vi "Servos Module Testing.vi"(0 "Stop Button":bool) -> ()   [LabVIEW 2015]
uses:
  <vilib>/FPGAPlugInAG/myRIO-1900/niLvFpga_Open_myRIO-1900.vi
  <vilib>/rvi/interface/common/dynamic/niFpgaDynamicAddResources.vi
  <vilib>/FPGAPlugInAG/Dynamic/niLvFpga_Run_Dynamic.vi
  <vilib>/FPGAPlugInAG/Dynamic/niLvFpga_Close_Dynamic.vi
  <vilib>/rvi/interface/nirviOpenFPGA/nirviOpenFPGA.xnode
  FPGA Bitfiles/PDMSMain_FPGATarget-Wi-Fi_Express2_Jo8xc+hAvHc.lvbitx
  FPGA/Express.vi
  <vilib>/rvi/interface/nirviMethod/nirviMethod.xnode
  <vilib>/rvi/interface/nirviCloseFPGA/nirviCloseFPGA.xnode
panel:
  in  "No. of Motors":enum16{"1", "2", "3", "4"}(ring)=enum."4"
  in  "Motor 4":enum16{"B", "S", "E", "C"}(ring)=enum."C"
  in  "Motor 3":enum16{"B", "S", "E", "C"}(ring)=enum."E"
  in  "Motor 2":enum16{"B", "S", "E", "C"}(ring)=enum."S"
  in  "Motor 1":enum16{"B", "S", "E", "C"}(ring)
  in  "Angle 4":u16=2250 min=500 max=2250
  in  "Angle 3":u16=2250 min=500 max=2250
  in  "Angle 2":u16=2250 min=500 max=2250
  in  "Angle 1":u16=2250 min=500 max=2250
  out "Error Out":errorcluster
  in  "Error In":errorcluster
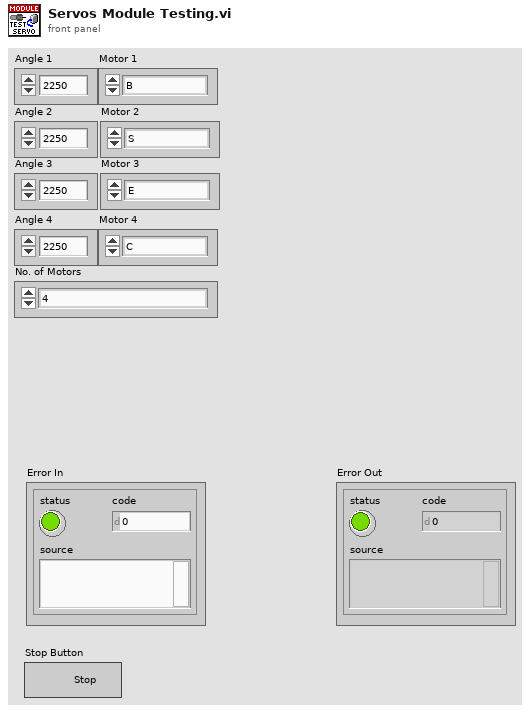
[diagram p1: front panel]
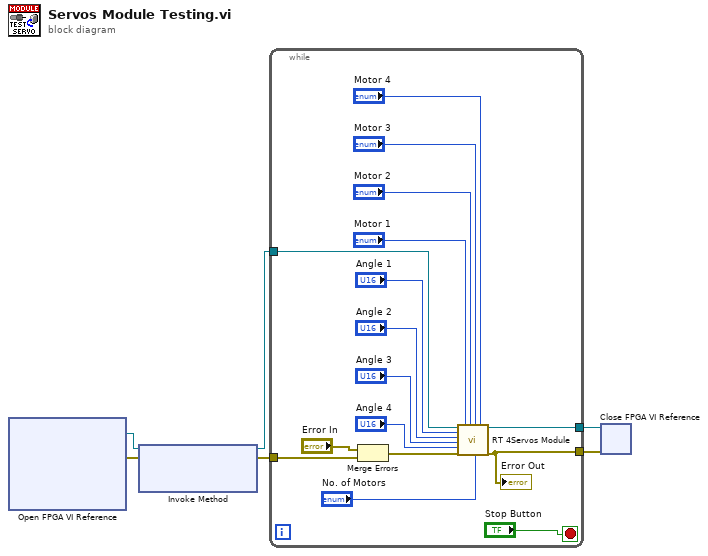
[diagram p0: block diagram]
diagram:
  n1 = xnode "Open FPGA VI Reference"() -> ("FPGA VI Reference Out"=w4:refnum<k20>, "error out"=w3:errorcluster)  [unwired: 2 in]
  n2 = xnode "Invoke Method"("FPGA VI Reference In"=w4, "error in"=w3) -> ("FPGA VI Reference Out"=w2:refnum<k20>, "error out"=w1:errorcluster)  [unwired: 1 in]
  n3 = while {
    tunnel: [w12] -> w6
    tunnel: [w11] -> w5
    tunnel: w2 -> [w8]
    tunnel: w1 -> [w7]
    stop <- "Stop Button" stop-if-true
    n4 = Merge Errors("Error In", w7) -> (w10:errorcluster)
    n5 = call "RT 4Servos Module.vi"("FPGA VI Reference In"=w8, "Angle 1"="Angle 1", "Angle 2"="Angle 2", "Angle 3"="Angle 3", "Angle 4"="Angle 4", "Error In"=w10, "Motor 1"="Motor 1", "Motor 2"="Motor 2", "Motor 3"="Motor 3", "No. of Motors"="No. of Motors", "Motor 4"="Motor 4") -> ("FPGA VI Reference Out"=w12:refnum<k20>, "Error Out"=w11:errorcluster)  [unwired: 7 in]
    "Error Out" <- w11
  }
  n6 = xnode "Close FPGA VI Reference"("FPGA VI Reference In"=w6, "error in"=w5) -> ()  [unwired: 1 out]
